vi "Clean FreeCache By Size.vi"(8 "error in (no error)":errorcluster, 10 "CacheSize":i32, 11 "MDPtrMgr in":refnum<class "MDPtrMgr.lvclass">) -> (0 "error out":errorcluster, 3 "MDPtrMgr out":refnum<class "MDPtrMgr.lvclass">)   [LabVIEW 2017, in "MDPtr.lvlib" / "MDPtrMgr.lvclass"]
uses:
  MDPtrMgr.lvclass
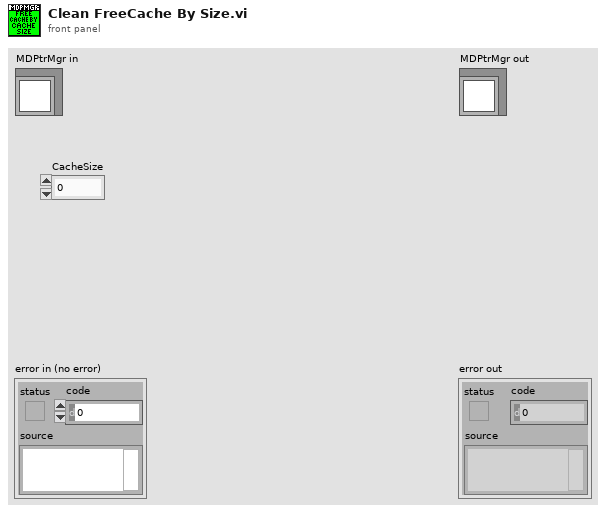
[diagram p1: front panel]
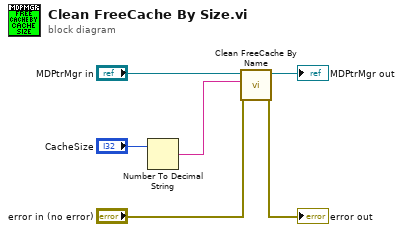
[diagram p0: block diagram]
diagram:
  n1 = Number To Decimal String(number="CacheSize") -> (decimal integer string=w4:string)  [unwired: 1 in]
  n2 = call "Clean FreeCache By Name.vi"("error in (no error)"="error in (no error)", "String"=w4, "MDPtrMgr in"="MDPtrMgr in") -> ("error out"=→"error out":errorcluster, "MDPtrMgr out"=→"MDPtrMgr out":refnum<class "MDPtrMgr.lvclass">)  [unwired: 7 in]
